vi "RT Main 7.vi"() -> ()   [LabVIEW 2019]
uses:
  <vilib>/FPGAPlugInAG/ELVIS III/niLvFpga_Open_ELVIS III.vi
  <vilib>/rvi/interface/common/dynamic/niFpgaDynamicAddResources.vi
  <vilib>/myRIO/Common/Instrument Driver Framework/Utilities/vis/FPGA Ref Manager.vi
  <vilib>/Utility/error.llb/Error Cluster From Error Code.vi
  <vilib>/myRIO/Common/Instrument Driver Framework/Utilities/vis/Ref Counter.vi
  <vilib>/rvi/errors/niLvFpgaAdjustHostInterfaceError.vi
  <vilib>/FPGAPlugInAG/Dynamic/niLvFpga_Close_Dynamic.vi
  <vilib>/rvi/interface/nirviOpenFPGA/nirviOpenFPGA.xnode
  FPGA Bitfiles/measurementpwmfr_FPGATarget_PWMMearsurement_UD6POuI2lT0.lvbitx
  <vilib>/rvi/interface/nirviReadWriteControl/nirviReadWriteControl.xnode
  <vilib>/rvi/interface/nirviCloseFPGA/nirviCloseFPGA.xnode
  <vilib>/myRIO/Instrument Drivers/Utilities/Utilities.lvlib
  NiFpgaLv.dll
  <vilib>/rvi/interface/Simulation/niFpgaSimulationCallBeginRW.vi
panel:
  out "双计数器法 2":dbl format="%#_15g"
  out "双计数器法":dbl format="%#_15g"
  out "error out":errorcluster
  in  "Stop":bool
  out "波形图表":dbl(graph)
  out "数值":dbl format="%#_16g"
  out "Error":dbl
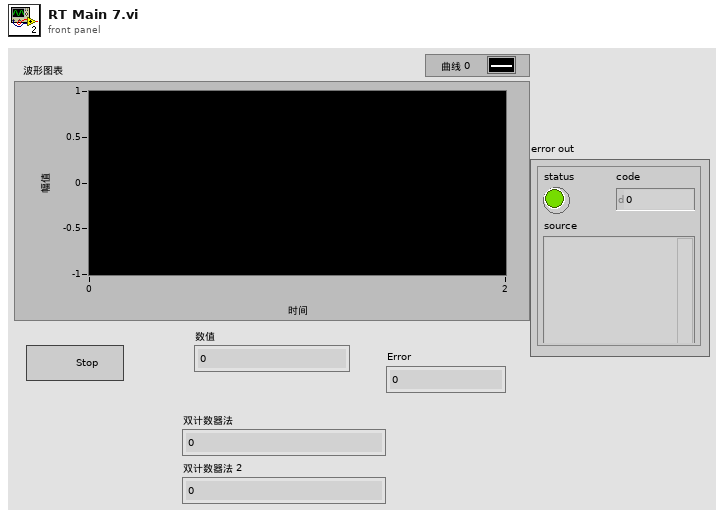
[diagram p1: front panel]
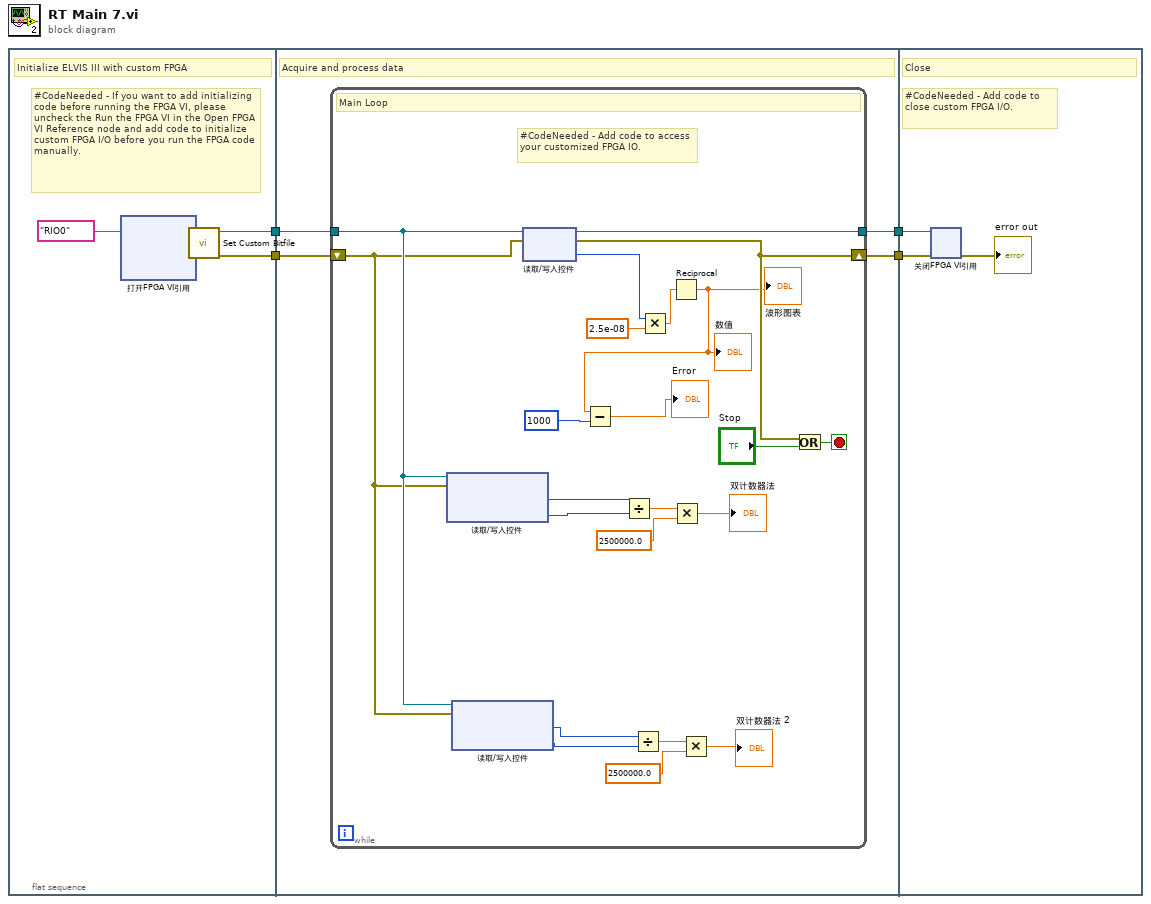
[diagram p0: block diagram]
diagram:
  n1 = flat-sequence {
    tunnel: [w6] -> w4
    tunnel: [w7] -> w3
    tunnel: w4 -> [w13]
    tunnel: w3 -> [w12]
    tunnel: [w11] -> w2
    tunnel: [w10] -> w1
    tunnel: w2 -> [w38]
    tunnel: w1 -> [w37]
    frame #0 {
      # "#CodeNeeded - If you want to add initializing code before running the FPGA VI, please uncheck the Run the FPGA VI in the Open FPGA VI Reference node and add code to initialize custom FPGA I/O before you run the FPGA code manually."
      # "Initialize ELVIS III with custom FPGA"
      n2 = xnode "打开FPGA VI引用"("资源名称"=tag "RIO0" ("resource name")) -> ("FPGA VI引用输出"=w8:refnum<k20>, "错误输出"=w9:errorcluster)  [unwired: 1 in]
      n3 = call <vilib>:"Set Custom Bitfile.vi"("error in (no error)"=w9, "Custom FPGA Reference In"=w8) -> ("error out"=w6:errorcluster, "Custom FPGA Reference Out"=w7:refnum<k20>)  [unwired: 8 in]
    }
    frame #1 {
      # "Acquire and process data"
      n4 = while {
        tunnel: w12 -> [w20]
        tunnel: [w33] -> w11
        shift-right: [w32] -> w10
        shift-left: w13 -> [w19]
        stop <- w34 stop-if-true
        # "#CodeNeeded - Add code to access your customized FPGA IO."
        # "Main Loop"
        n5 = xnode "读取/写入控件"("FPGA VI引用输入"=w20, "错误输入"=w19) -> ("被测信号个数 2"=w23:u32, "时钟信号个数 2"=w21:u32)  [unwired: 2 out]
        n6 = xnode "读取/写入控件"("FPGA VI引用输入"=w20, "错误输入"=w19) -> ("被测信号个数 3"=w15:u32, "时钟信号个数 3"=w16:u32)  [unwired: 2 out]
        n7 = xnode "读取/写入控件"("FPGA VI引用输入"=w20, "错误输入"=w19) -> ("FPGA VI引用输出"=w33:refnum<k20>, "错误输出"=w32:errorcluster, "x-1"=w24:u32)
        n8 = Divide(x=w23, y=w21) -> (x/y=w26:dbl)
        n9 = Divide(x=w15, y=w16) -> (x/y=w17:dbl)
        n10 = Multiply(x=w24, y=2.5e-08) -> (x*y=w31:dbl)
        n11 = Reciprocal(x=w31) -> (1/x=w29:dbl)
        "波形图表" <- w29
        "数值" <- w29
        n12 = Subtract(x=w29, y=u32 1000) -> (x-y=→"Error":dbl)
        n13 = Multiply(x=w26, y=2500000.0) -> (x*y=→"双计数器法":dbl)
        n14 = Multiply(x=w17, y=2500000.0) -> (x*y=→"双计数器法 2":dbl)
        n15 = Or(x=w32, y="Stop") -> (x .or. y?=w34:bool)
      }
    }
    frame #2 {
      # "#CodeNeeded - Add code to close custom FPGA I/O."
      # "Close"
      n16 = xnode "关闭FPGA VI引用"("FPGA VI引用输入"=w38, "错误输入"=w37) -> ("错误输出"=→"error out":errorcluster)
    }
  }
